vi "Compare.vi"(1 "Transaction y":refnum<class "Transaction.lvclass">, 2 "Transaction x":refnum<class "Transaction.lvclass">) -> (0 "Equal?":bool)   [LabVIEW 2018, in "Transaction.lvclass"]
uses:
  Transaction.lvclass
  Transaction.lvclass/Transaction.ctl
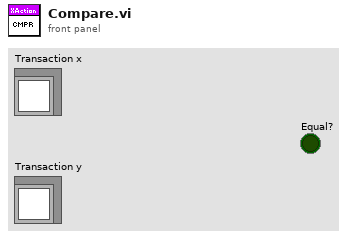
[diagram p1: front panel]
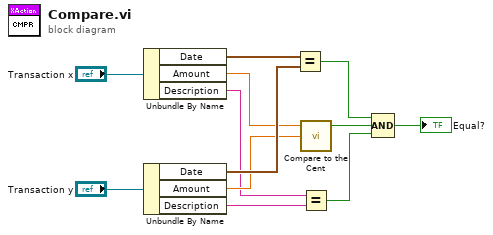
[diagram p0: block diagram]
diagram:
  n1 = Unbundle By Name("Transaction x") -> ("Date"=w11:timestamp, "Amount"=w9:dbl, "Description"=w6:string)
  n2 = Unbundle By Name("Transaction y") -> ("Date"=w10:timestamp, "Amount"=w8:dbl, "Description"=w5:string)
  n3 = Equal?(x=w11, y=w10) -> (x = y?=w12:bool)
  n4 = call "Compare to the Cent.vi"("Dollar y"=w8, "Dollar x"=w9) -> ("x = y?"=w7:bool)  [unwired: 3 in]
  n5 = Equal?(x=w6, y=w5) -> (x = y?=w4:bool)
  n6 = Compound Arithmetic op=AND(w12, w7, w4) -> (→"Equal?":bool)
